vi "Iso8601FileName.vi"(5 "UTC":bool, 7 "TimeStamp":timestamp, 10 "Extension (.log)":string=".log", 11 "Prefix ('')":string) -> (3 "FileName":string)   [LabVIEW 2022 SP3, in "DateTime.lvlib"]
uses:
  DateTime.lvlib
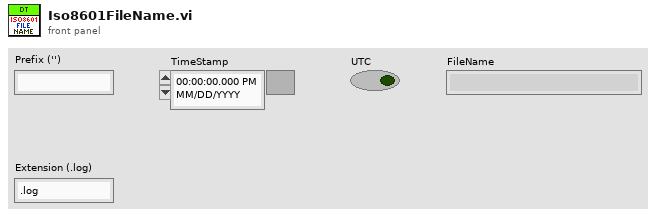
[diagram p1: front panel]
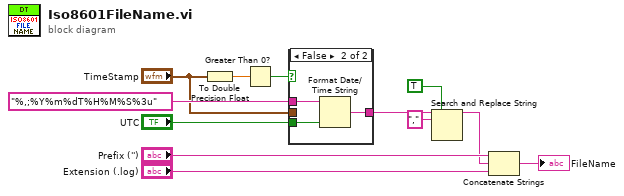
[diagram p0: block diagram]
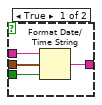
[diagram p2: hidden frame]
diagram:
  n1 = To Double Precision Float(number="TimeStamp") -> (double precision float=w2:dbl)
  n2 = Greater Than 0?(x=w2) -> (x > 0?=w1:bool)
  n3 = case shown="False" w1 {
    tunnel: "%,;%Y%m%dT%H%M%S%3u" ("time format string (%c)") -> [w16 w19]
    tunnel: [w15 w18] -> w11
    tunnel: "UTC" -> [w14 w17]
    tunnel: "TimeStamp" -> [w13 _]
    frame True {
      n4 = Format Date/Time String(time format string (%c)=w16, seconds (now)=w13, UTC format=w14) -> (date/time string=w15:string)
    }
    frame False {
      n5 = Format Date/Time String(time format string (%c)=w19, UTC format=w17) -> (date/time string=w18:string)  [unwired: 1 in]
    }
  }
  n6 = Search and Replace String(replace all?=TRUE ("replace all? (F)"), input string=w11, search string=",") -> (result string=w6:string)  [unwired: 5 in, 3 out]
  n7 = Concatenate Strings("Prefix ('')", w6, "Extension (.log)") -> (→"FileName":string)
